vi "探头窗口-2-网络版.vi"() -> ()   [LabVIEW 2017]
panel:
  out "引用-监测模式？":refnum<vi>
  in  "外部停止命令？":bool=TRUE
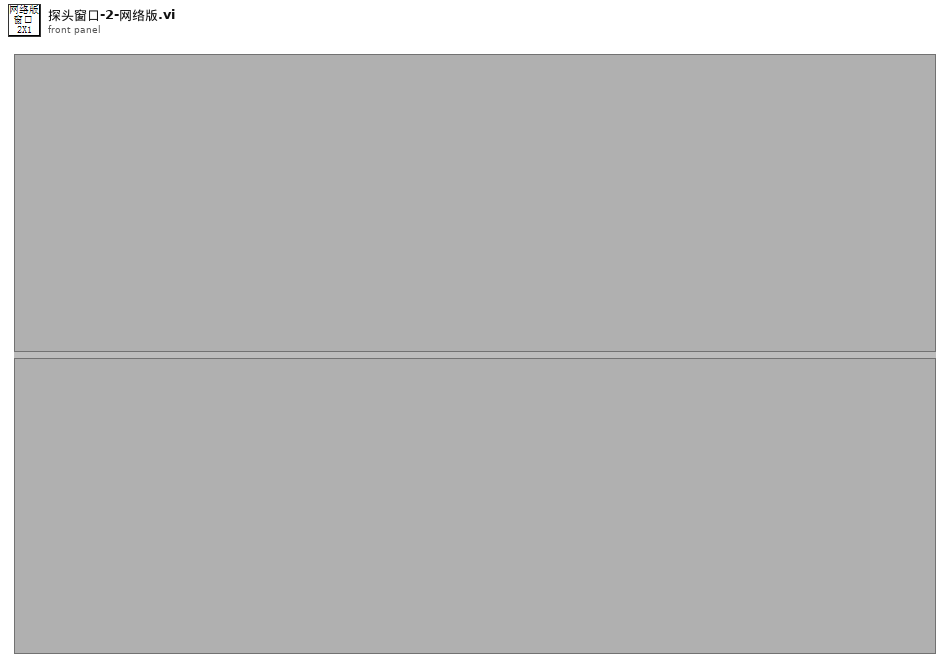
[diagram p1: front panel]
types:
  T1 = enum32{"Invalid", "Standard", "Closed", "Hidden", "Minimized", "Maximized"}
  T2 = typedef "eventvkey.ctl" = enum16{"ASCII", "Enter", "Return", "Shift", "Ctrl", "Alt", "Cmd", "Opt", "Caps", "NumLock", "Clear", "Break", "Up", "Down", "Left", "Right", "Insert", "Delete", "Home", "End", "PageUp", "PageDown", "Escape", "Help", "Pause", "ScrollLock", "F1", "F2", "F3", "F4", "F5", "F6", "F7", "F8", "F9", "F10", "F11", "F12", "F13", "F14", "F15", "F16", "F17", "F18", "F19", "F20", "F21", "F22", "F23", "F24", "Play", "VolumeUp", "VolumeDown", "Mute", "Two Byte Char"}
  T3 = typedef "探头属性.ctl" = cluster{"探头地址与信息":T4, "测量值":T7, "限值":T8, "探头状态":T9, "累积记录":T10, "报警方式":T11}
  T4 = typedef "探测器信息.ctl" = cluster{"网络地址":string, "名称":string, "备注":string, "累积剂量":dbl, "累积限值":dbl, "硬件剂量率限值":T5, "剂量率限值1":dbl, "剂量率限值2":dbl, "报警方式":T6}
  T5 = typedef "探头剂量率限值选择.ctl" = enum16{"一级限值", "二级限值"}
  T6 = typedef "报警方式选择.ctl" = enum16{"常报警", "自动静音", "手动静音"}
  T7 = typedef "测量值.ctl" = cluster{"时间":timestamp, "数值":dbl}
  T8 = typedef "剂量率限值.ctl" = cluster{"限值1":dbl, "限值2":dbl, "探头限值":T5}
  T9 = typedef "探头状态.ctl" = enum16{"正常", "离线", "禁用", "一级报警", "二级报警", "累积报警"}
  T10 = typedef "单条累积记录.ctl" = cluster{"起始时间":timestamp, "结束时间":timestamp, "累积剂量":dbl}
  T11 = typedef "报警方式.ctl" = cluster{"报警方式":T6, "延迟计时":u16, "报警中？":bool}
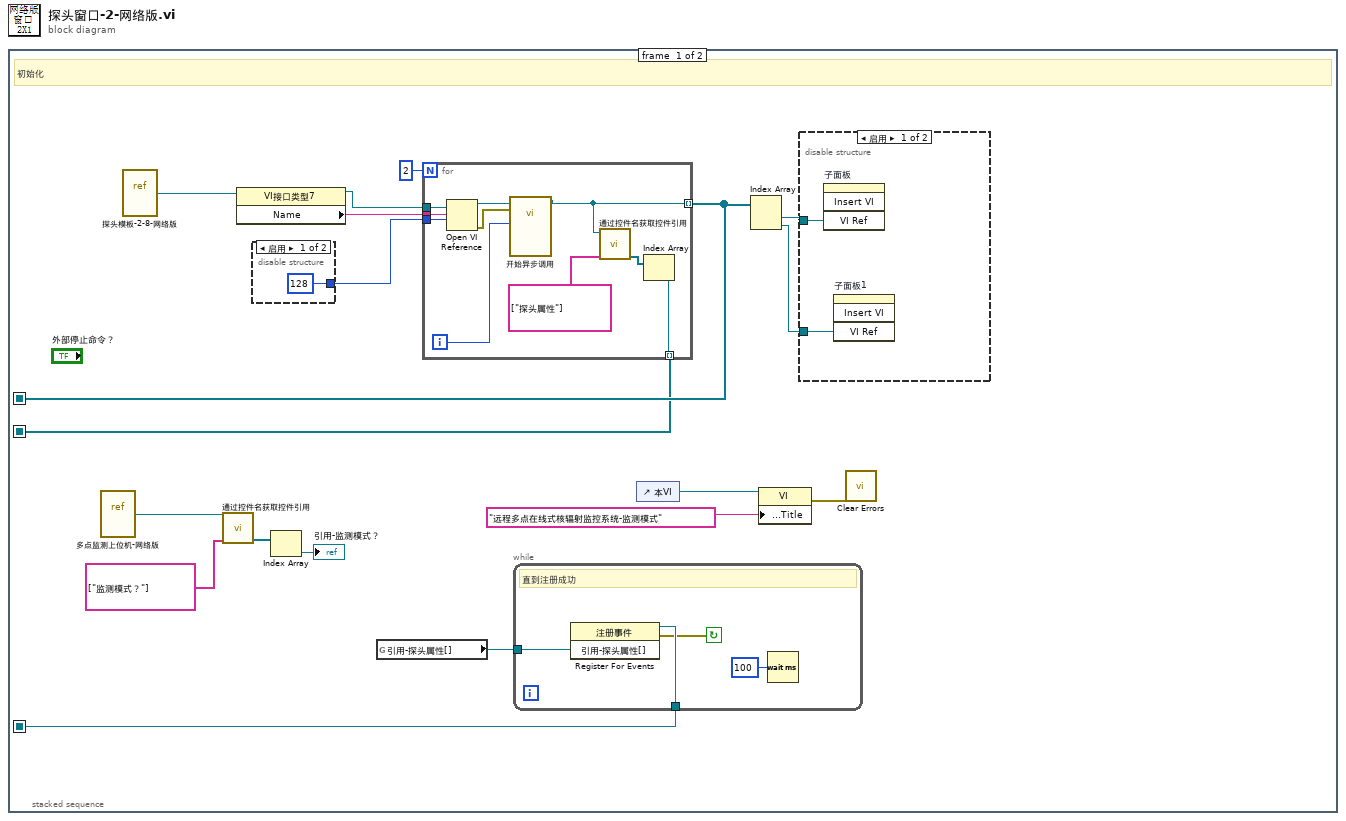
[diagram p0: block diagram]
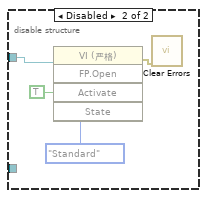
[diagram p2: hidden frame]
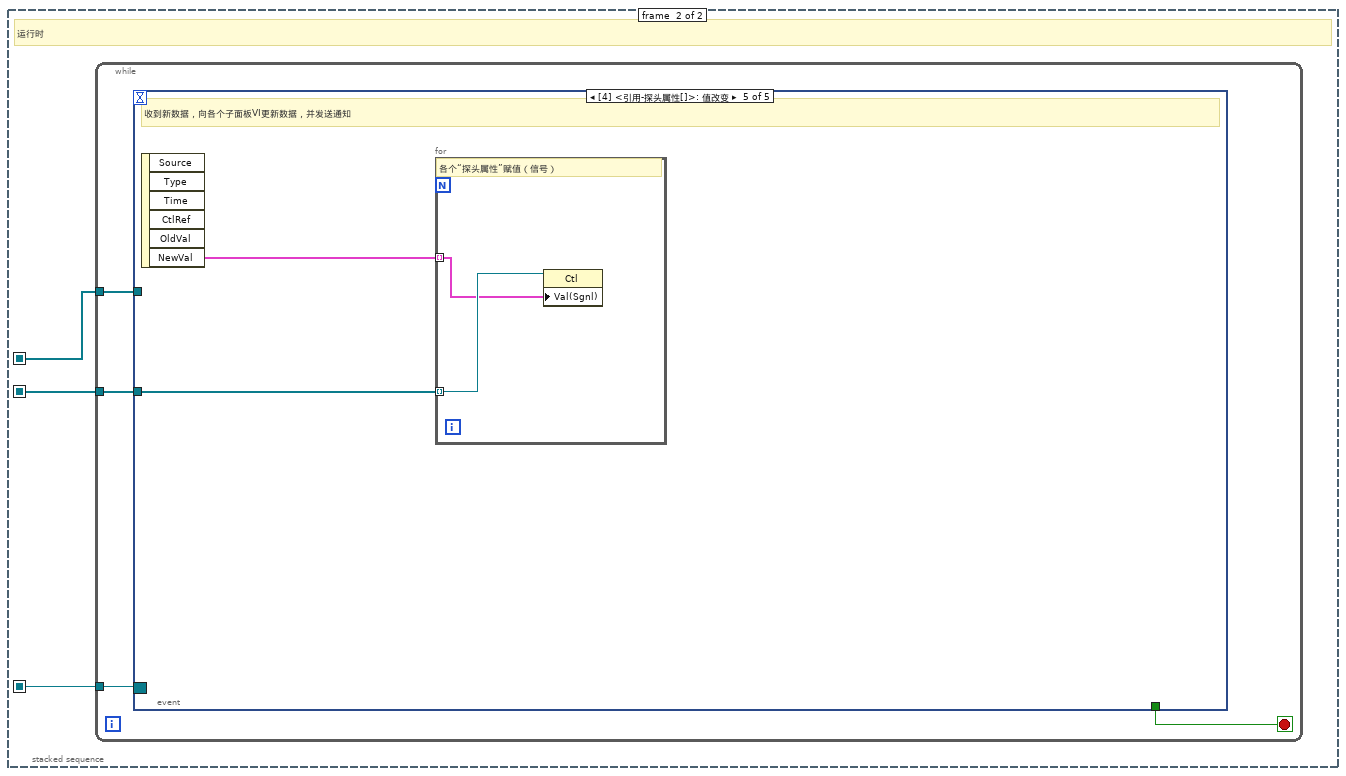
[diagram p4: hidden frame]
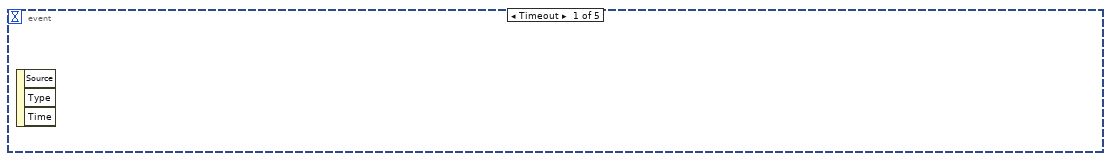
[diagram p5: hidden frame]
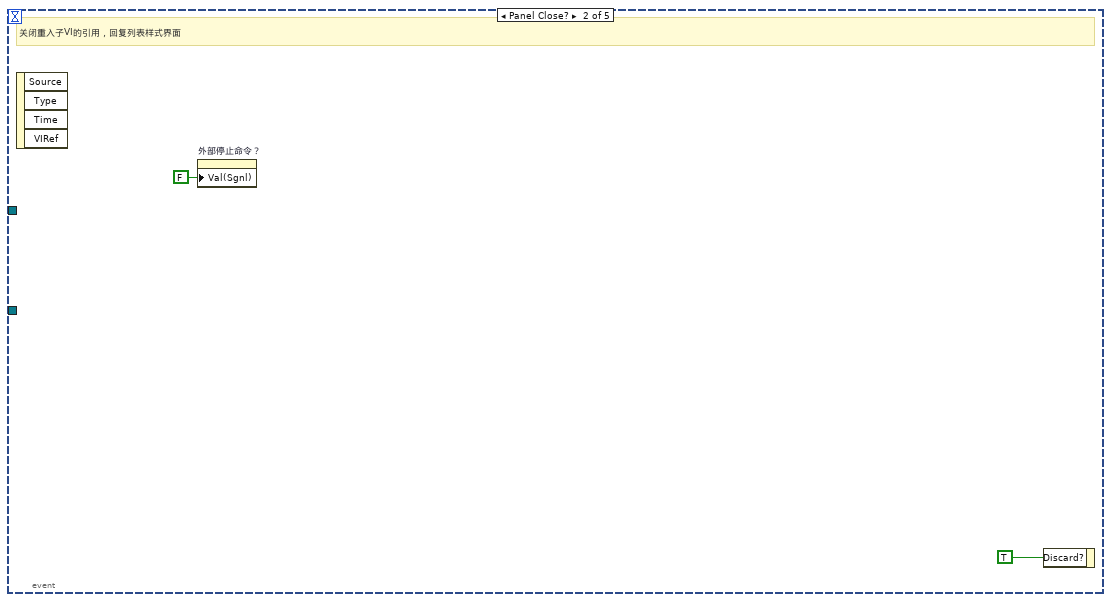
[diagram p6: hidden frame]
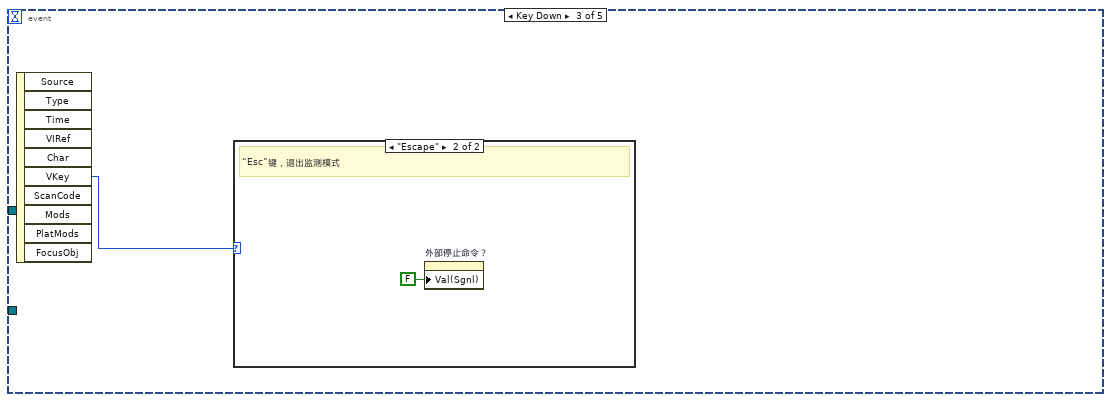
[diagram p7: hidden frame]
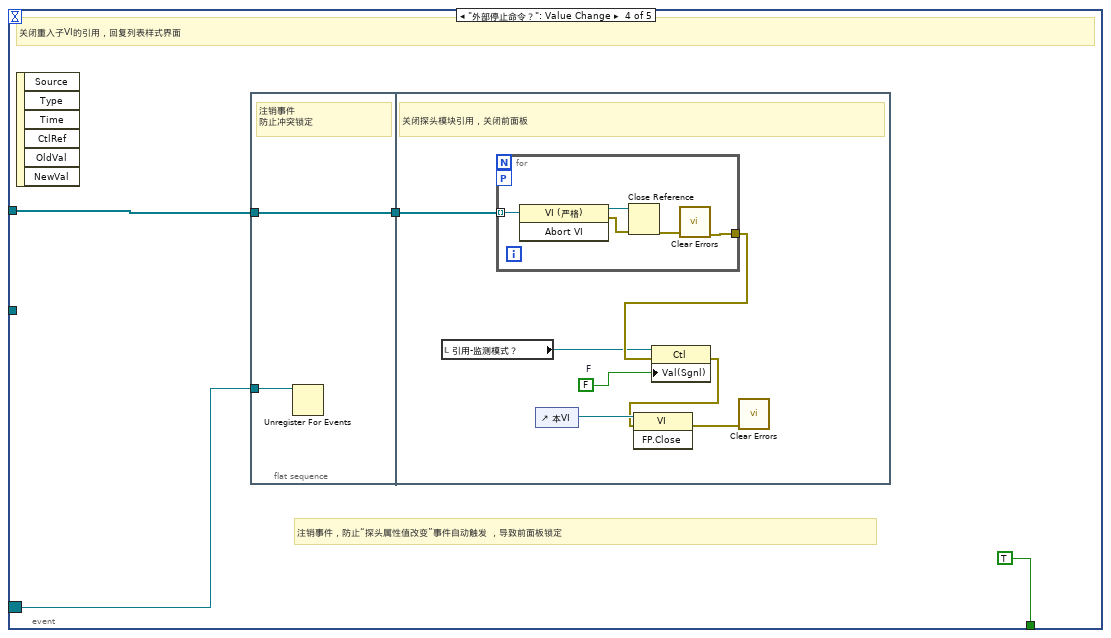
[diagram p9: hidden frame]
diagram:
  n1 = stacked-sequence {
    seq-local: [w15 _] -> [_ w42]
    seq-local: [w11 _] -> [_ w41]
    seq-local: [w2 _] -> [_ w40]
    frame #0 {
      # "初始化"
      n2 = vi-ref "多点监测上位机-网络版.vi"() -> (w7:refnum<vi>)
      n3 = vi-ref "探头模板-2-8-网络版.vi"() -> (w18:refnum<vi>)
      n4 = call "通过控件名获取控件引用.vi"("控件名数组"=string[] ["监测模式？"], "VI引用"=w7) -> ("控件引用输出"=w5:refnum<vi>[])  [unwired: 7 in, 2 out]
      n5 = property class="VI接口类型7"(reference=w18) -> (reference out=w3:refnum<vi>, "Name"=w17:string)  [unwired: 1 in, 1 out]
      n6 = disable-structure shown="启用" {
        disable-tunnel: [128 ("选项") _] -> w16
        frame Enabled {
        }
        frame Disabled {
        }
      }
      n7 = Index Array(array=w5) -> (element=→"引用-监测模式？":refnum<vi>)  [unwired: 1 in]
      n8 = global read "全局变量-35点监测.vi" "引用-探头属性[]"() -> (w1:refnum<vi>)
      n9 = for "For循环" {
        N: 2 -> [_]
        tunnel: w17 -> [w39]
        tunnel: w16 -> [w38]
        tunnel: w3 -> [w37]
        tunnel: [w32] -> w15 mode=indexing
        tunnel: [w34] -> w11 mode=indexing
        i -> [w31]
        n10 = Open VI Reference(type specifier VI Refnum (for type only)=w37, vi path=w39, options=w38) -> (vi reference=w33:refnum<vi>, error out=w30:errorcluster)  [unwired: 3 in]
        n11 = call-by-ref "开始异步调用"(reference=w33, error in=w30, "探头序号"=w31) -> (reference out=w32:refnum<vi>)  [unwired: 11 in, 1 out]
        n12 = call "通过控件名获取控件引用.vi"("控件名数组"=string[] ["探头属性"], "VI引用"=w32) -> ("控件引用输出"=w35:refnum<vi>[])  [unwired: 7 in, 2 out]
        n13 = Index Array(array=w35) -> (element=w34:refnum<vi>)  [unwired: 1 in]
      }
      n14 = while {
        tunnel: w1 -> [w22]
        tunnel: [w21] -> w2
        stop <- w20 continue-if-true
        # "直到注册成功"
        n15 = register-events(w22) -> (reference out=w21:refnum<event-registration>, error out=w20:errorcluster)  [unwired: 2 in]
        n16 = Wait (ms)(milliseconds to wait=u32 100 ("等待时间（毫秒）")) -> ()  [unwired: 1 out]
      }
      n17 = control-ref of="本VI"() -> (w10:refnum<vi>)
      n18 = Index Array(array=w15) -> (element #1=w14:refnum<vi>, element #2=w13:refnum<vi>)  [unwired: 2 in]
      n19 = property class="VI"(reference=w10, "Front Panel.Title"="远程多点在线式核辐射监控系统-监测模式" ("前面板窗口:标题")) -> (error out=w8:errorcluster)  [unwired: 1 in, 1 out]
      n20 = disable-structure shown="启用" {
        disable-tunnel: w14 -> [w24 w28]
        disable-tunnel: w13 -> [w23 _]
        frame Enabled {
          n21 = invoke on="子面板" class="子面板" method="Insert VI"("VI Ref"=w24) -> ()  [unwired: 3 in, 4 out]
          n22 = invoke on="子面板1" class="SubPnl" method="Insert VI"("VI Ref"=w23) -> ()  [unwired: 3 in, 4 out]
        }
        frame Disabled {
          n23 = invoke class="VI (严格)" method="FP.Open"(reference=w28, "Activate"=TRUE ("激活？"), "State"=T1."Standard" ("状态")) -> (error out=w25:errorcluster)  [unwired: 2 in, 4 out]
          n24 = call <vilib>:"Clear Errors.vi"("error in (no error)"=w25) -> ()  [unwired: 5 in, 2 out]
        }
      }
      n25 = call <vilib>:"Clear Errors.vi"("error in (no error)"=w8) -> ()  [unwired: 5 in, 2 out]
    }
    frame #1 {
      # "运行时"
      n26 = while {
        tunnel: w42 -> [w45]
        tunnel: w41 -> [w44]
        tunnel: w40 -> [w43]
        stop <- w46 stop-if-true
        n27 = event shown="[4] <引用-探头属性[]>: 值改变" {
          selector: w43 -> [_ _ _ w51 _]
          dyn-events: _ -> [_ _ _ _ _]
          timeout: _ -> [_ _ _ _ _]
          tunnel: [_ _ _ TRUE ("放弃？") _] -> w46
          tunnel: w45 -> [_ _ _ w53 _]
          tunnel: w44 -> [_ _ _ _ w70]
          event Timeout {
            n28 = event-data() -> ()  [unwired: 1 in, 3 out]
          }
          event Panel Close? {
            # "关闭重入子VI的引用，回复列表样式界面"
            n29 = event-data() -> ()  [unwired: 1 in, 4 out]
            n30 = property on="外部停止命令？" class="Bool (严格)"("Val(Sgnl)"=FALSE ("值(信号)")) -> ()  [unwired: 2 in, 2 out]
            n31 = event-data("Discard?"=TRUE ("放弃？")) -> ()  [unwired: 1 in, 1 out]
          }
          event Key Down {
            n32 = event-data() -> ("VKey"=w49:T2)  [unwired: 1 in, 9 out]
            n33 = case shown="\"Escape\"" w49 {
              frame "ASCII", Default {
              }
              frame "Escape" {
                # "“Esc”键，退出监测模式"
                n34 = property on="外部停止命令？" class="Bool (严格)"("Val(Sgnl)"=FALSE ("值(信号)")) -> ()  [unwired: 2 in, 2 out]
              }
            }
          }
          event "外部停止命令？": Value Change {
            # "注销事件，防止“探头属性值改变”事件自动触发 ，导致前面板锁定"
            # "关闭重入子VI的引用，回复列表样式界面"
            n35 = event-data() -> ()  [unwired: 1 in, 6 out]
            n36 = flat-sequence {
              tunnel: w53 -> [w56]
              tunnel: [w56] -> w52
              tunnel: w51 -> [w55]
              tunnel: w52 -> [w63]
              frame #0 {
                # "注销事件\n防止冲突锁定"
                n37 = Unregister For Events(event registration refnum=w55) -> ()  [unwired: 1 in, 1 out]
              }
              frame #1 {
                w62 = FALSE  # F
                # "关闭探头模块引用，关闭前面板"
                n38 = local read "引用-监测模式？"() -> (w57:refnum<vi>)
                n39 = for "For循环" {
                  tunnel: w63 -> [w68] mode=indexing
                  workers-P: _ -> [_]
                  tunnel: [w64] -> w60
                  n40 = invoke class="VI (严格)" method="Abort VI"(reference=w68) -> (reference out=w67:refnum<vi>, error out=w66:errorcluster)  [unwired: 2 in, 1 out]
                  n41 = Close Reference(reference=w67, error in (no error)=w66) -> (error out=w65:errorcluster)
                  n42 = call <vilib>:"Clear Errors.vi"("error in (no error)"=w65) -> ("error out"=w64:errorcluster)  [unwired: 5 in, 1 out]
                }
                n43 = control-ref of="本VI"() -> (w61:refnum<vi>)
                n44 = property class="Ctl"(reference=w57, error in=w60, "Val(Sgnl)"=w62) -> (error out=w59:errorcluster)  [unwired: 1 out]
                n45 = invoke class="VI" method="FP.Close"(reference=w61, error in=w59) -> (error out=w58:errorcluster)  [unwired: 1 in, 2 out]
                n46 = call <vilib>:"Clear Errors.vi"("error in (no error)"=w58) -> ()  [unwired: 5 in, 2 out]
              }
            }
          }
          event Value Change {
            # "收到新数据，向各个子面板VI更新数据，并发送通知"
            n47 = event-data() -> ("NewVal"=w69:T3[])  [unwired: 1 in, 5 out]
            n48 = for "For循环" {
              tunnel: w70 -> [w72] mode=indexing
              tunnel: w69 -> [w71] mode=indexing
              # "各个“探头属性”赋值（信号）"
              n49 = property class="Ctl"(reference=w72, "Val(Sgnl)"=w71) -> ()  [unwired: 1 in, 2 out]
            }
          }
        }
      }
    }
  }
